vi "simpleExample.vi"() -> ()   [LabVIEW 2019]
uses:
  <vilib>/regexp/Match Regular Expression.xnode
panel:
  out "Resistance":dbl(knob) scale=0.0..0.0002 scale format="%#_2p"
  in  "time per reading (ms)":u32
  in  "stop":bool
  out "Temp":dbl
  out "Resistance":dbl format="%#_6p"
  out "error out":errorcluster
  in  "Mode":T1(ring)
  in  "VISA resource name":refnum<visa-resource-name>
  # "Change the range by double\n clicking the max value on the scale"
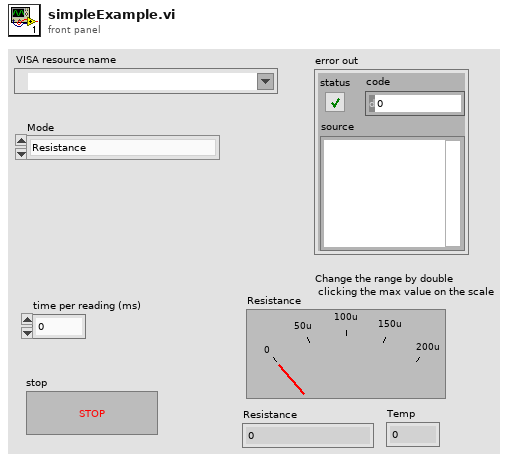
[diagram p1: front panel]
types:
  T1 = enum16{"Resistance", "Resistance and Temp", "Low Power Resistance", "Low Power Resisance and Temp", "Temp"}
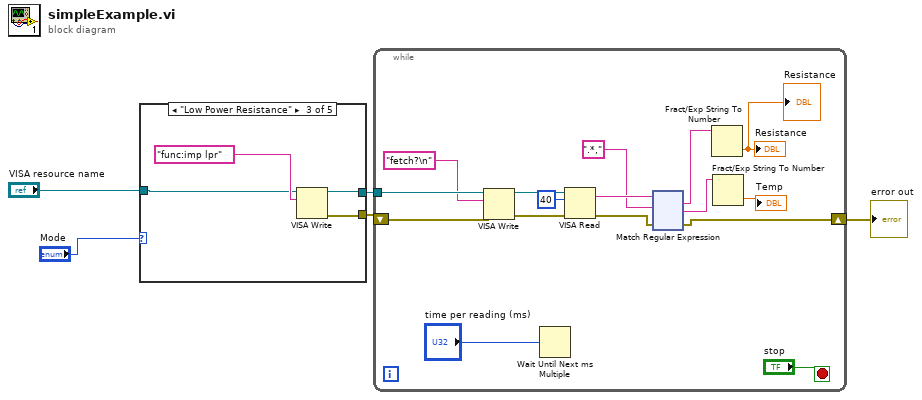
[diagram p0: block diagram]
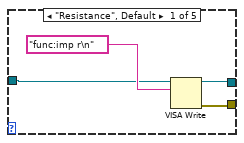
[diagram p2: hidden frame]
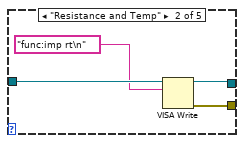
[diagram p3: hidden frame]
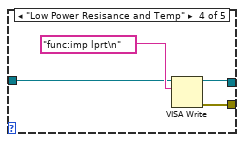
[diagram p4: hidden frame]
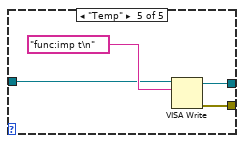
[diagram p5: hidden frame]
diagram:
  n1 = case shown="\"Low Power Resistance\"" "Mode" {
    tunnel: "VISA resource name" -> [w8 w13 w16 w20 w24]
    tunnel: [w7 w11 w15 w19 w23] -> w3
    tunnel: [w6 w10 w14 w18 w22] -> w2
    frame "Resistance", Default {
      n2 = VISA Write(VISA resource name=w8, write buffer="func:imp r\n") -> (VISA resource name out=w7:refnum<visa-resource-name>, error out=w6:errorcluster)  [unwired: 1 in, 1 out]
    }
    frame "Resistance and Temp" {
      n3 = VISA Write(VISA resource name=w13, write buffer="func:imp rt\n") -> (VISA resource name out=w11:refnum<visa-resource-name>, error out=w10:errorcluster)  [unwired: 1 in, 1 out]
    }
    frame "Low Power Resistance" {
      n4 = VISA Write(VISA resource name=w16, write buffer="func:imp lpr") -> (VISA resource name out=w15:refnum<visa-resource-name>, error out=w14:errorcluster)  [unwired: 1 in, 1 out]
    }
    frame "Low Power Resisance and Temp" {
      n5 = VISA Write(VISA resource name=w20, write buffer="func:imp lprt\n") -> (VISA resource name out=w19:refnum<visa-resource-name>, error out=w18:errorcluster)  [unwired: 1 in, 1 out]
    }
    frame "Temp" {
      n6 = VISA Write(VISA resource name=w24, write buffer="func:imp t\n") -> (VISA resource name out=w23:refnum<visa-resource-name>, error out=w22:errorcluster)  [unwired: 1 in, 1 out]
    }
  }
  n7 = while {
    tunnel: w3 -> [w41]
    shift-right: [w32] -> w1
    shift-left: w2 -> [w40]
    stop <- "stop" stop-if-true
    n8 = VISA Write(VISA resource name=w41, write buffer="fetch?\n", error in (no error)=w40) -> (VISA resource name out=w38:refnum<visa-resource-name>, error out=w37:errorcluster)  [unwired: 1 out]
    n9 = Wait Until Next ms Multiple(millisecond multiple="time per reading (ms)") -> ()  [unwired: 1 out]
    n10 = VISA Read(VISA resource name=w38, byte count=u32 40, error in (no error)=w37) -> (read buffer=w35:string, error out=w34:errorcluster)  [unwired: 2 out]
    n11 = xnode "Match Regular Expression"("input string"=w35, "regular expression"=".*,", "error in"=w34) -> ("whole match"=w31:string, "after match"=w30:string, "error out"=w32:errorcluster)  [unwired: 3 in, 2 out]
    n12 = Fract/Exp String To Number(string=w31) -> (number=→"Resistance" →"Resistance":dbl)  [unwired: 3 in, 1 out]
    n13 = Fract/Exp String To Number(string=w30) -> (number=→"Temp":dbl)  [unwired: 3 in, 1 out]
  }
  "error out" <- w1
